vi "Slice String.vi"(5 "Include String[j] (false)":bool, 7 "Subset (i:j)":string, 8 "String":string) -> (1 "Substring (String[i:j])":string)   [LabVIEW 2015]
doc: "Returns a <B>substring</B>, specified by <B>subset</B>, from <B>string</B>. \n\nSlice String.vi was originally written to emulate the slice notation of Python. (See below for extended capabilities.) In Python, a slice is a subset of elements in a list and a string is a list of characters. If you want to access one character in the string (or one element in any list), you'd use the list name and the index value:\n\n<B>substring</B> = <B>string</B>[i]\n\nTo get multple contiguous characters, use the slice i:j notation in place of the single index:\n\n<B>substring</B> = <B>string</B>[i:j]\n\nCharacters (elements) are assigned to the output starting at the first index value, and continuing up to, but not including, the last value.\n\nIn this notation, i and j are integers.\nThe first character in <B>string</B> has index zero.\nIf i is ommitted it is assumed to be zero and <B>substring</B>contains the leftmost characters of <B>string</B>.\nIf j is ommitted it is assumed to be length(string) and <B>substring</B>contains the rightmost characters of <B>string</B>.\nIf i or j are negative numbers they are assumed to be referenced from the end of the string.\n\nIn the LabVIEW implementation, the range of the slice is expressed in the string variable <B>subset</B> as \"i:j\".\n\nSlice String.vi has now been extended to allow the (optional) inclusion of the last value as well (for those who are used to the closed interval syntax) by wiring a TRUE constant to the fourth terminal. (Only two of the examples below, in boldface, are affected.)\n\nExamples:\n\nIf <B>string</B> = \"MyString\" \nfor <B>include string[j]</B> = FALSE (default) / for <B>include string[j]</B> = TRUE\n\nstring[2:] = \"String\" string[2:] = \"String\"\nstring[:3] = \"MyS\" string[:3] = \"<B>MySt</B>\"\nstring[-1] = \"g\" string[-1] = \"g\"\nstring[4] = \"r\" string[4] = \"r\"\nstring[-4:-2] = \"ri\" string[-4:-2] = \"<B>rin</B>\""
panel:
  # "Slice String.vi\n\nThis VI uses indices to extract a substring from a string.\n\nPlease visit http://www.OpenG.org to learn about the\nOpen Source LabVIEW software movement.\n\nNOTICE -- YOU MUST LEAVE THIS NOTICE IN PLACE.  PER THE TERMS OF THE LICENSE BELOW, YOU MAY SUBLICENSE THIS SOFTWARE \nIN ANY WAY THAT DOES NOT CONFLICT WITH THIS LICENSE.\n\n### BSD License (http://www.opensource.org/licenses/bsd-license.php) Begin ###\n \nCopyright (c) 2002, Jim Kring <jim@jimkring.com>\nCopyright (c) 2002, Cal-Bay Systems, Inc. <info@calbay.com>\nCopyright (c) 2004, Paul F. Sullivan <Paul@SULLutions.com>\nCopyright (c) 2011, Jonathon Green <jg@jgcode.net>\n\nAll rights reserved.\n\nRedistribution and use in source and binary forms, with or without modification, are permitted provided that the following conditions are met:\n\n    * Redistributions of source code must retain the above copyright notice, this list of conditions and the following disclaimer.\n    * Redistributions in binary form must reproduce the above copyright notice, this list of conditions and the following disclaimer in the \n       documentation and/or other materials provided with the distribution.\n    * Neither the name of SciWare, James Kring, Inc., nor the names of its contributors may be used to endorse or promote products derived \n       from this software without specific prior written permission.\n\nTHIS SOFTWARE IS PROVIDED BY THE COPYRIGHT HOLDERS AND CONTRIBUTORS \"AS IS\" AND ANY EXPRESS OR IMPLIED WARRANTIES, \nINCLUDING, BUT NOT LIMITED TO, THE IMPLIED WARRANTIES OF MERCHANTABILITY AND FITNESS FOR A PARTICULAR PURPOSE ARE \nDISCLAIMED. IN NO EVENT SHALL THE COPYRIGHT OWNER OR CONTRIBUTORS BE LIABLE FOR ANY DIRECT, INDIRECT, INCIDENTAL,\n SPECIAL, EXEMPLARY, OR CONSEQUENTIAL DAMAGES (INCLUDING, BUT NOT LIMITED TO, PROCUREMENT OF SUBSTITUTE GOODS OR \nSERVICES; LOSS OF USE, DATA, OR PROFITS; OR BUSINESS INTERRUPTION) HOWEVER CAUSED AND ON ANY THEORY OF LIABILITY, \nWHETHER IN CONTRACT, STRICT LIABILITY, OR TORT (INCLUDING NEGLIGENCE OR OTHERWISE) ARISING IN ANY WAY OUT OF THE USE \nOF THIS SOFTWARE, EVEN IF ADVISED OF THE POSSIBILITY OF SUCH DAMAGE.\n\n### BSD License End ###"
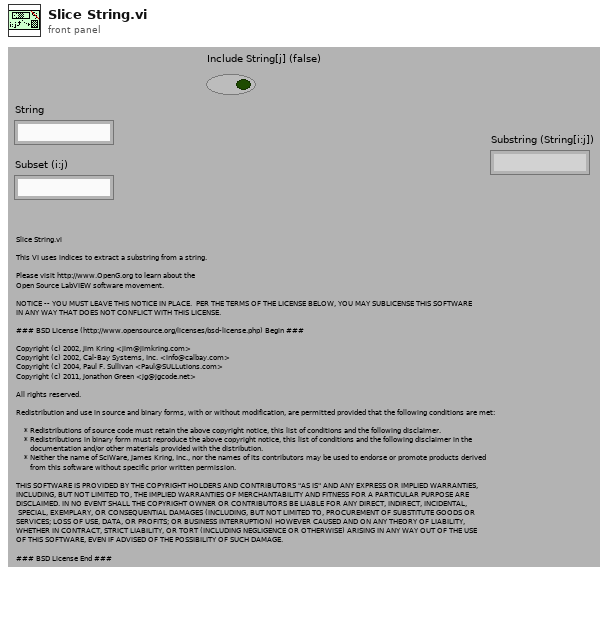
[diagram p1: front panel]
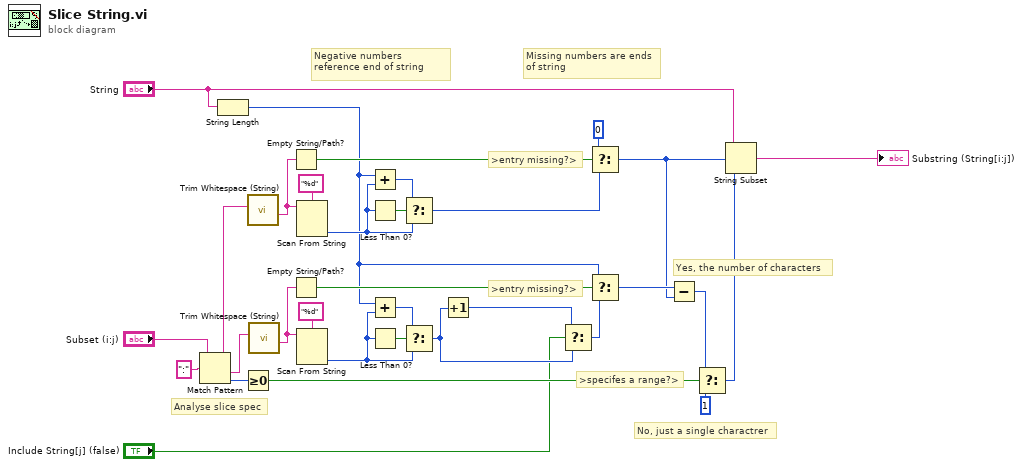
[diagram p0: block diagram]
diagram:
  # "Analyse slice spec"
  # "Negative numbers reference end of string"
  # "Missing numbers are ends of string"
  # "Yes, the number of characters"
  # "No, just a single charactrer"
  # ">entry missing?>"
  # ">entry missing?>"
  # ">specifes a range?>"
  n1 = Match Pattern ("Analyze slice spec.")(string="Subset (i:j)", regular expression=":" ("search string/char (-)")) -> (before substring=w4:string, after substring=w2:string, offset past match=w12:i32)  [unwired: 1 in, 1 out]
  n2 = String Length(string="String") -> (length=w17:i32)
  n3 = Greater Or Equal To 0?(x=w12) -> (x >= 0?=w11:bool)
  n4 = call "Trim Whitespace (String).vi"("String in"=w4) -> ("String out"=w3:string)  [unwired: 6 in]
  n5 = call "Trim Whitespace (String).vi"("String in"=w2) -> ("String out"=w1:string)  [unwired: 6 in]
  n6 = Empty String/Path?(string/path=w3) -> (empty?=w23:bool)
  n7 = Empty String/Path?(string/path=w1) -> (empty?=w18:bool)
  n8 = Scan From String(format string="%d" ("Format String"), input string=w3) -> (output 1=w28:i32)  [unwired: 3 in, 3 out]
  n9 = Scan From String(format string="%d" ("Format String"), input string=w1) -> (output 1=w22:i32)  [unwired: 3 in, 3 out]
  n10 = Add(x=w17, y=w28) -> (x+y=w27:i32)
  n11 = Less Than 0?(x=w28) -> (x < 0?=w26:bool)
  n12 = Add(x=w17, y=w22) -> (x+y=w21:i32)
  n13 = Less Than 0?(x=w22) -> (x < 0?=w20:bool)
  n14 = Select(t=w27, s=w26, f=w28) -> (s? t:f=w9:i32)
  n15 = Select(t=w21, s=w20, f=w22) -> (s? t:f=w6:i32)
  n16 = Increment ("Include limit.")(x=w6) -> (x+1=w8:i32)
  n17 = Select(t=w8, s="Include String[j] (false)", f=w6) -> (s? t:f=w7:i32)
  n18 = Select(t=0 ("length"), s=w23, f=w9) -> (s? t:f=w15:i32)
  n19 = Select(t=w17, s=w18, f=w7) -> (s? t:f=w16:i32)
  n20 = Subtract ("Yes, the number of characters.")(x=w16, y=w15) -> (x-y=w14:i32)
  n21 = Select(t=w14, s=w11, f=1 ("No, just a single character.")) -> (s? t:f=w13:i32)
  n22 = String Subset(string="String", offset (0)=w15, length (rest)=w13) -> (substring=→"Substring (String[i:j])":string)
